vi "Initialize Plugin Settings.vi"(8 "error in (no error)":errorcluster, 10 "Plugins":refnum<class "Plugin.lvclass">[](array[class]), 11 "Dispatcher in":refnum<class "Dispatcher Thread.lvclass">) -> (0 "error out":errorcluster, 3 "Dispatcher out":refnum<class "Dispatcher Thread.lvclass">)   [LabVIEW 2017, in "DSF Core.lvlib" / "Dispatcher Thread.lvclass"]
uses:
  Dispatcher Thread.lvclass
  Plugin/Plugin.lvclass
  Plugin Settings.ctl
  Thread Pool/Plugin Interface Pool.lvclass
  Plugin/Plugin.lvclass/Plugin.ctl
  Transfer Group/Transfer Group.lvclass/Transfer Group.ctl
  Dispatcher Thread.lvclass/Dispatcher Thread.ctl
  Transfer Group/Transfer Group.lvclass
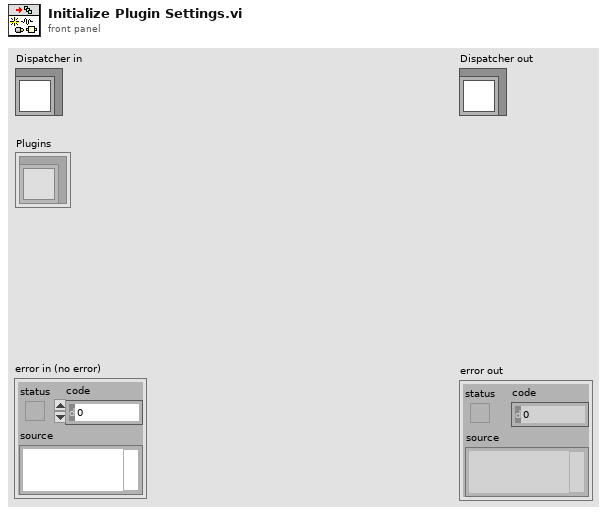
[diagram p1: front panel]
types:
  T1 = typedef "DSF Core.lvlib/Dispatcher Thread.lvclass/Plugin Settings.ctl" = cluster{"Transfer Group threads":i32[], "Plugin Thread Pool":refnum<class "Plugin Interface Pool.lvclass">}
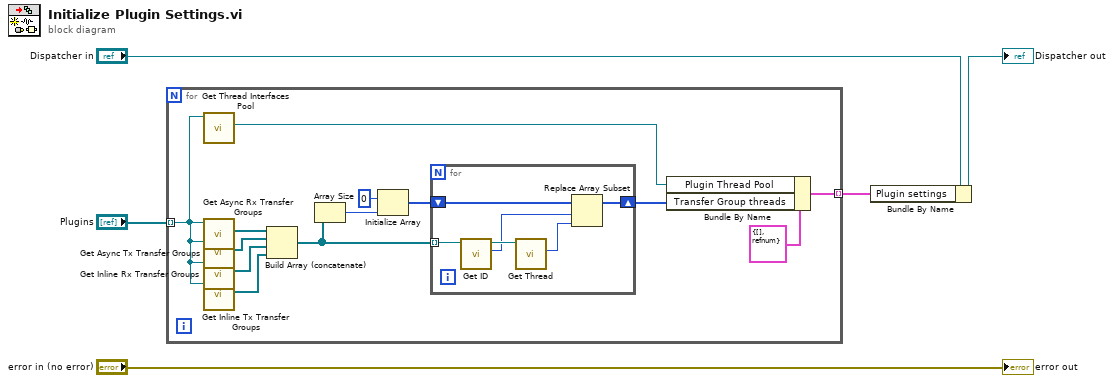
[diagram p0: block diagram]
diagram:
  n1 = for {
    tunnel: "Plugins" -> [w7] mode=indexing
    tunnel: [w8] -> w3 mode=indexing
    n2 = call "Get Thread Interfaces Pool.vi"("Plugin in"=w7) -> ("Plugin Interfaces Pool"=w6:refnum<class "Plugin Interface Pool.lvclass">)  [unwired: 9 in, 1 out]
    n3 = call "Get Async Rx Transfer Groups.vi"("Plugin in"=w7) -> ("Async Rx Transfer Groups"=w16:refnum<class "Transfer Group.lvclass">[])  [unwired: 9 in, 1 out]
    n4 = call "Get Async Tx Transfer Groups.vi"("Plugin in"=w7) -> ("Async Tx Transfer Groups"=w17:refnum<class "Transfer Group.lvclass">[])  [unwired: 9 in, 1 out]
    n5 = call "Get Inline Rx Transfer Groups.vi"("Plugin in"=w7) -> ("Inline Rx Transfer Groups"=w15:refnum<class "Transfer Group.lvclass">[])  [unwired: 9 in, 1 out]
    n6 = call "Get Inline Tx Transfer Groups.vi"("Plugin in"=w7) -> ("Inline Tx Transfer Groups"=w18:refnum<class "Transfer Group.lvclass">[])  [unwired: 9 in, 1 out]
    n7 = Build Array (concatenate)(w16, w17, w15, w18) -> (w12:refnum<class "Transfer Group.lvclass">[])
    n8 = Array Size(array=w12) -> (size(s)=w14:i32)
    n9 = Initialize Array(0 ("element"), w14) -> (w11:i32[])
    n10 = for {
      tunnel: w12 -> [w24] mode=indexing
      shift-right: [w19] -> w9
      shift-left: w11 -> [w22]
      n11 = call "Get ID.vi"("Transfer Group in"=w24) -> ("id"=w21:i32, "Transfer Group out"=w23:refnum<class "Transfer Group.lvclass">)  [unwired: 9 in]
      n12 = call "Get Thread.vi"("Transfer Group in"=w23) -> ("thread"=w20:i32)  [unwired: 9 in, 1 out]
      n13 = Replace Array Subset(array=w22, new element=w20, index=w21) -> (w19:i32[])
    }
    n14 = Bundle By Name(cluster=T1 {"Transfer Group threads"=[], "Plugin Thread Pool"=refnum} ("plugins settings"), "Plugin Thread Pool"=w6, "Transfer Group threads"=w9) -> (w8:T1)
  }
  n15 = Bundle By Name(cluster="Dispatcher in", "Plugin settings"=w3) -> (→"Dispatcher out":refnum<class "Dispatcher Thread.lvclass">)
  "error out" <- "error in (no error)"
